vi "MALT IOPS.vi"() -> ()   [LabVIEW 2018, in "AltonTech MALT200817.lvlib"]
uses:
  AltonTech MALT200817.lvlib
panel:
  out "IOPS":u32
  out "Total Time":u32
  out "data out":string
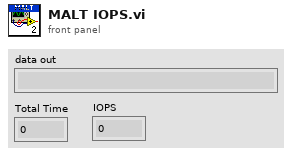
[diagram p1: front panel]
types:
  T1 = enum16{"Standard", "Buffered", "CRLF", "Immediate"}
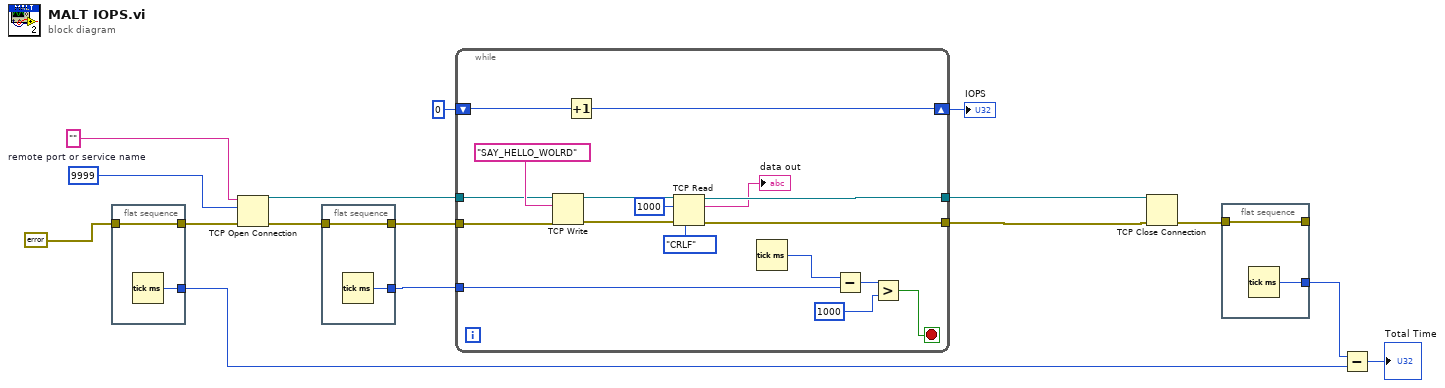
[diagram p0: block diagram]
diagram:
  w12 = u16 9999  # remote port or service name
  n1 = flat-sequence {
    tunnel: errorcluster {"status"=FALSE, "code"=0, "source"=""} ("error in (no error)") -> [w18]
    tunnel: [w18] -> w13
    tunnel: [w17] -> w11
    frame #0 {
      n2 = Tick Count (ms)() -> (millisecond timer value=w17:u32)
    }
  }
  n3 = TCP Open Connection(address="", remote port or service name=w12, error in (no error)=w13) -> (connection ID=w3:refnum<k5>, error out=w6:errorcluster)  [unwired: 2 in]
  n4 = flat-sequence {
    tunnel: w6 -> [w20]
    tunnel: [w20] -> w5
    tunnel: [w19] -> w4
    frame #0 {
      n5 = Tick Count (ms)() -> (millisecond timer value=w19:u32)
    }
  }
  n6 = while {
    tunnel: [w37] -> w16
    tunnel: [w36] -> w7
    tunnel: w5 -> [w29]
    tunnel: w4 -> [w27]
    tunnel: w3 -> [w26]
    shift-right: [w23] -> w2
    shift-left: u32 0 ("x") -> [w24]
    stop <- w25 stop-if-true
    n7 = TCP Write(connection ID=w26, data in="SAY_HELLO_WOLRD", error in (no error)=w29) -> (connection ID out=w35:refnum<k5>, error out=w30:errorcluster)  [unwired: 1 in, 1 out]
    n8 = Increment(x=w24) -> (x+1=w23:u32)
    n9 = TCP Read(connection ID=w35, bytes to read=1000, error in (no error)=w30, 7:T1."CRLF" ("mode (standard)")) -> (connection ID out=w37:refnum<k5>, data out=→"data out":string, error out=w36:errorcluster)  [unwired: 1 in]
    n10 = Tick Count (ms)() -> (millisecond timer value=w28:u32)
    n11 = Subtract(x=w28, y=w27) -> (x-y=w22:u32)
    n12 = Greater?(x=w22, y=u32 1000 ("x")) -> (0:w25:bool)
  }
  "IOPS" <- w2
  n13 = TCP Close Connection(connection ID=w16, error in (no error)=w7) -> (error out=w9:errorcluster)  [unwired: 1 in, 1 out]
  n14 = flat-sequence {
    tunnel: w9 -> [w39]
    tunnel: [w39] -> _
    tunnel: [w38] -> w8
    frame #0 {
      n15 = Tick Count (ms)() -> (millisecond timer value=w38:u32)
    }
  }
  n16 = Subtract(x=w8, y=w11) -> (x-y=→"Total Time":u32)
